vi "Axis Page.vi"() -> ()   [LabVIEW 2017, in "3D Plot.lvclass"]
uses:
  <vilib>/Math Plots/3D Math Plots/3D Plot/3D Plot/3D Plot.lvclass
  <vilib>/Math Plots/3D Math Plots/3D Plot/3D Plot/Typedef/Axis Property.ctl
  <vilib>/Math Plots/3D Math Plots/3D Plot/3D Plot/Typedef/Caption Property.ctl
  <vilib>/Math Plots/3D Math Plots/3D Plot/3D Plot/Typedef/Label Property.ctl
  <vilib>/Math Plots/3D Math Plots/3D Plot/3D Plot/Typedef/Range Property.ctl
  <vilib>/Math Plots/3D Math Plots/3D Plot/3D Plot/Typedef/Range Clusters.ctl
  <vilib>/Math Plots/3D Math Plots/3D Plot/3D Plot/Typedef/Grid Property.ctl
  <vilib>/Math Plots/3D Math Plots/3D Plot/3D Plot/Typedef/Tick Property.ctl
  <vilib>/Math Plots/3D Math Plots/3D Plot/3D Plot/Typedef/Dialog State.ctl
  <vilib>/Math Plots/3D Math Plots/3D Plot/3D Plot/Typedef/Temp Scene State.ctl
  <vilib>/Math Plots/3D Math Plots/3D Plot/3D Plot/Typedef/Temp Scene Property Action.ctl
panel:
  in  "Active Axis":u16(ring) caption="Active axis" items=["X Axis", "Y Axis", "Z Axis"]
  in  "Range Logarithm":bool caption="Range logarithm"
  in  "Marker Size":u16=1 caption="Size" min=1 step=1
  in  "Name Label Size":u16=1 caption="Size" min=1 step=1
  in  "Name Label Text":string caption="Text"
  in  "Marker Color":u32(colorbox) caption="Color"
  in  "Name Label Color":u32(colorbox) caption="Color"
  in  "Major Grid Color":u32(colorbox) caption="Major grid color"
  in  "Minor Grid Color":u32(colorbox) caption="Minor grid color"
  in  "Major Tick Color":u32(colorbox) caption="Major tick color"
  in  "Minor Tick Color":u32(colorbox) caption="Minor tick color"
  in  "Name Label Normal Visible":bool caption="Name label normal visible"
  in  "Name Label Opposite Visible":bool caption="Name label opposite visible"
  in  "Marker Normal Visible":bool caption="Marker normal visible"
  in  "Marker Opposite Visible":bool caption="Marker opposite visible"
  in  "Major Grid Visible":bool caption="Major grid visible"
  in  "Minor Grid Visible":bool caption="Minor grid visible"
  in  "Major Tick Visible":bool caption="Major tick visible"
  in  "Minor Tick Visible":bool caption="Major tick visible"
  in  "Major Tick Count":u16=1 caption="Major tick count" min=1 step=1
  in  "Minor Tick Count":u16=1 caption="Minor tick count" min=1 step=1
  in  "Range Auto Scale":bool caption="Range auto scale"
  in  "Range Inverted":bool caption="Range inverted"
  in  "Range Minimum":sgl caption="Minimum"
  in  "Range Maximum":sgl caption="Maximum"
  in  "Event Registration":refnum<event-registration>
  out "Axis Property Out":T1
  in  "Axis Property In":T1
  # "Axis"
  # "Name Label"
  # "Marker"
  # "Range"
  # "Grid"
  # "Tick"
  # "Tick Spacing"
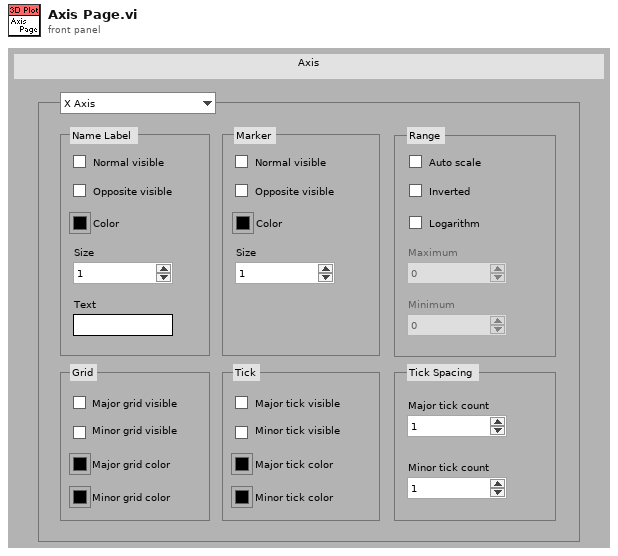
[diagram p1: front panel]
types:
  T1 = typedef "3D Plot.lvclass/Axis Property.ctl" = cluster{"Caption Property":T2, "Label Property":T3, "Range Property":T4, "Grid Property":T6, "Ticks Property":T7}
  T2 = typedef "3D Plot.lvclass/Caption Property.ctl" = cluster{"Show Caption":cluster{"Show Normal X Caption":bool, "Show Normal Y Caption":bool, "Show Normal Z Caption":bool, "Show Opposite X Caption":bool, "Show Opposite Y Caption":bool, "Show Opposite Z Caption":bool}, "Caption Color":cluster{"Caption Color X":u32, "Caption Color Y":u32, "Caption Color Z":u32}, "Caption Size":cluster{"Caption Size X":u16, "Caption Size Y":u16, "Caption Size Z":u16}, "Caption String":cluster{"Caption X":string, "Caption Y":string, "Caption Z ":string}}
  T3 = typedef "3D Plot.lvclass/Label Property.ctl" = cluster{"Show Label":cluster{"Show Normal X Label":bool, "Show Normal Y Label":bool, "Show Normal Z Label":bool, "Show Opposite X Label":bool, "Show Opposite Y Label":bool, "Show Opposite Z Label":bool}, "Label Color":cluster{"Label Color X":u32, "Label Color Y":u32, "Label Color Z":u32}, "Label Size":cluster{"Label Size X":u16, "Label Size Y":u16, "Labe Size Z":u16}}
  T4 = typedef "3D Plot.lvclass/Range Property.ctl" = cluster{"Range Cluster":T5, "Auto Range":cluster{"Auto Range X":bool, "Auto Range Y":bool, "Auto Range Z":bool}, "Inverted":cluster{"Inverted X":bool, "Inverted Y":bool, "Inverted Z":bool}, "Logarithm":cluster{"Logarithm X":bool, "Logarithm Y":bool, "Logarithm Z":bool}}
  T5 = typedef "3D Plot.lvclass/Range Clusters.ctl" = cluster{"X Range":cluster{"Max X":sgl, "Min X":sgl}, "Y Range":cluster{"Max Y":sgl, "Min Y":sgl}, "Z Range":cluster{"Max Z":sgl, "Min Z":sgl}}
  T6 = typedef "3D Plot.lvclass/Grid Property.ctl" = cluster{"Major Grid Visible":cluster{"Draw Major Grid X":bool, "Draw Major Grid Y":bool, "Draw Major Grid Z":bool}, "Major Grid Color":cluster{"Major Grid Color X":u32, "Major Grid Color Y":u32, "Major Grid Color Z":u32}, "Minor Grid Visible":cluster{"Draw Minor Grid X":bool, "Draw Minor Grid Y":bool, "Draw Minor Grid Z":bool}, "Minor Grid Color":cluster{"Minor Grid Color X":u32, "Minor Grid Color Y":u32, "Minor Grid Color Z":u32}}
  T7 = typedef "3D Plot.lvclass/Tick Property.ctl" = cluster{"Major Tick Visible":cluster{"Draw Major Tick X":bool, "Draw Major Tick Y":bool, "Draw Major Tick Z":bool}, "Major Tick Color":cluster{"Major Tick Color X":u32, "Major Tick Color Y":u32, "Major Tick Color Z":u32}, "Major Count":cluster{"Major Count X":u16, "Major Count Y":u16, "Major Count Z":u16}, "Minor Tick Visible":cluster{"Draw Minor Tick X":bool, "Draw Minor Tick Y":bool, "Draw Minor Tick Z":bool}, "Minor Tick Color":cluster{"Minor Tick Color X":u32, "Minor Tick Color Y":u32, "Minor Tick Color Z":u32}, "Minor Count":cluster{"Minor Count X":u16, "Minor Count Y":u16, "Minor Count Z":u16}}
  T8 = typedef "3D Plot.lvclass/Dialog State.ctl" = enum16{"Initialize", "Read Porperty", "Write Property", "Idle", "Exit"}
  T9 = typedef "3D Plot.lvclass/Axis Property Array Element.ctl" = cluster{"Caption":string, "Caption Size":u16, "Caption Color":u32, "Show Normal Caption":bool, "Show Opposite Caption":bool, "Label Size":u16, "Label Color":u32, "Show Normal Label":bool, "Show Opposite Label":bool, "Auto Range":bool, "Inverted":bool, "Logarithm":bool, "Max":sgl, "Min":sgl, "Draw Major Grid":bool, "Major Grid Color":u32, "Draw Minor Grid":bool, "Minor Grid Color":u32, "Major Count":u16, "Draw Major Tick":bool, "Major Tick Color":u32, "Minor Count":u16, "Draw Minor Tick":bool, "Minor Tick Color":u32}
  T10 = typedef "3D Plot.lvclass/Temp Scene State.ctl" = enum16{"Create", "Update Scene", "Get Plot Representation", "Destory"}
  T11 = typedef "3D Plot.lvclass/Temp Scene Property Action.ctl" = enum16{"Graph Property", "Light Property", "Axis Property", "Value Pair Property", "Format Property", "Cursor Property", "Plot Specific Property"}
  T12 = typedef "3D Plot.lvclass/Multiplot Representation.ctl" = cluster{"Plot Represention Array":T13[], "Max Range":T5}
  T13 = typedef "3D Plot.lvclass/Plot Representation.ctl" = cluster{"Plot ID":i32, "Plot Range":T5, "Mesh Data":T14, "Dimension":cluster{"X Dimension":i32, "Y Dimension":i32}, "Ramp Range":T5}
  T14 = typedef "3D Plot.lvclass/Mesh Data.ctl" = cluster{"Index Array":u32[], "Vertex Array":cluster{"X":sgl, "Y":sgl, "Z":sgl}[], "Normal Array":cluster{"X":sgl, "Y":sgl, "Z":sgl}[], "Color Index Array":i32[]}
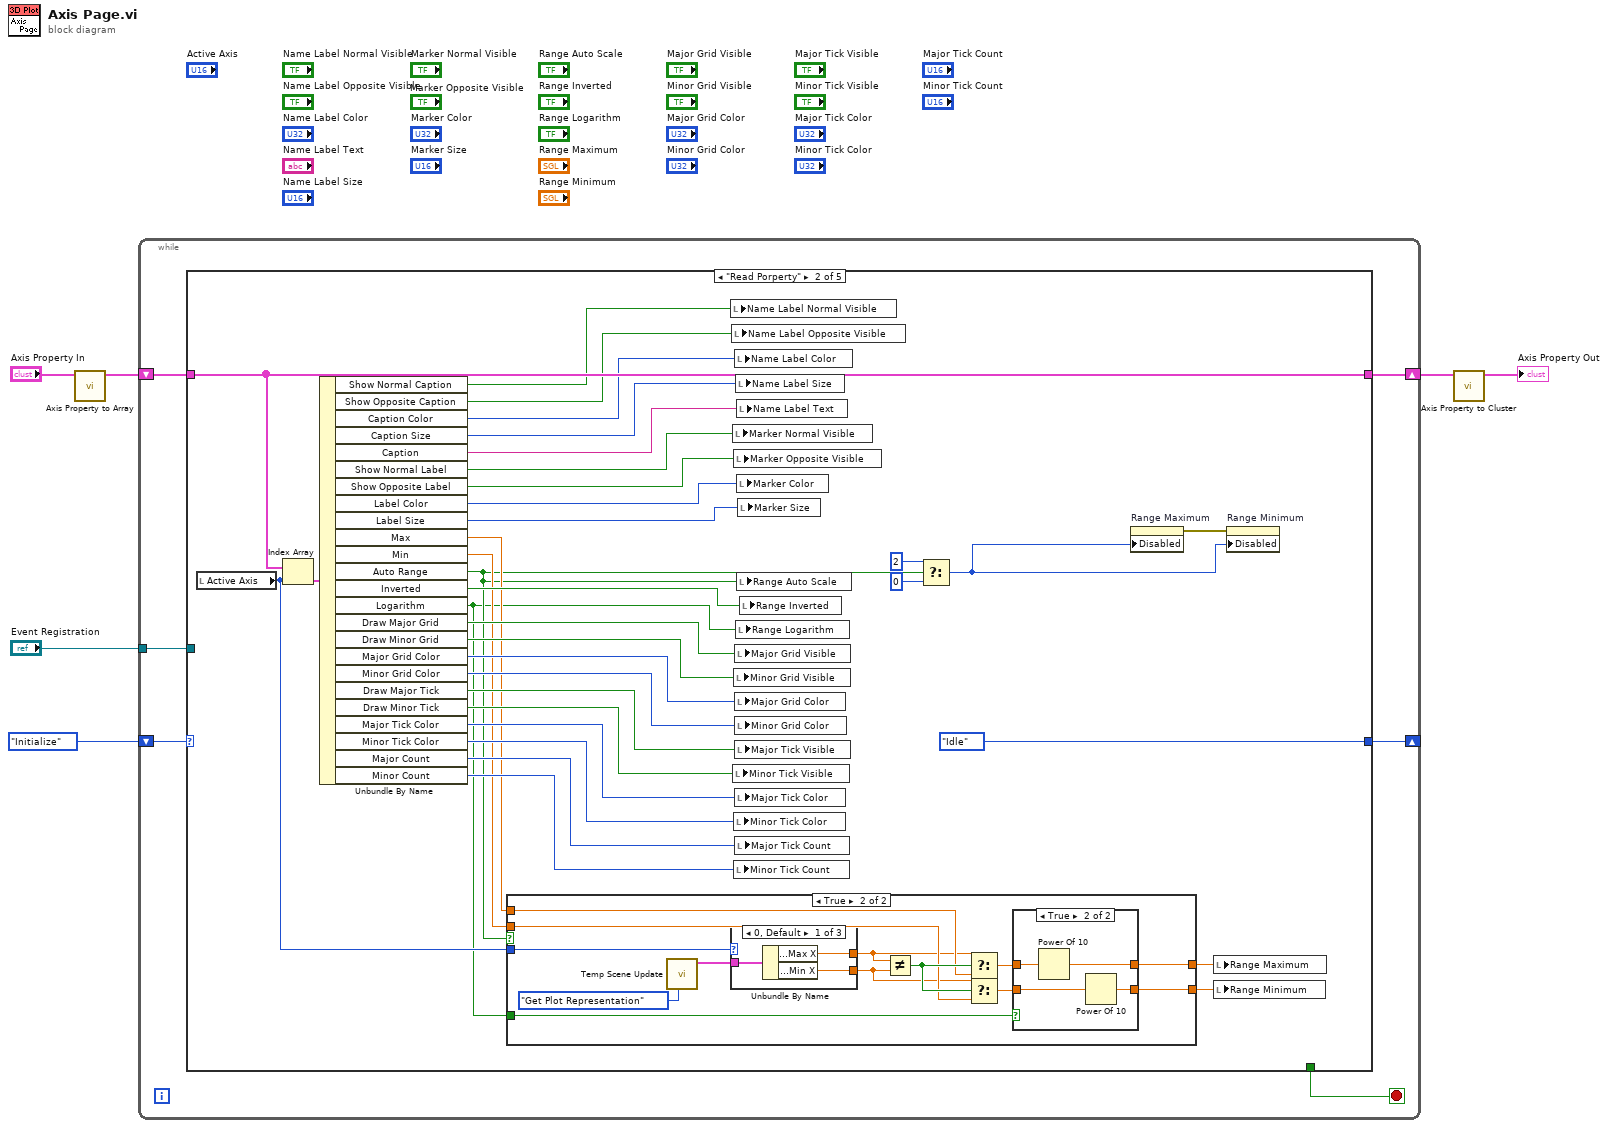
[diagram p0: block diagram]
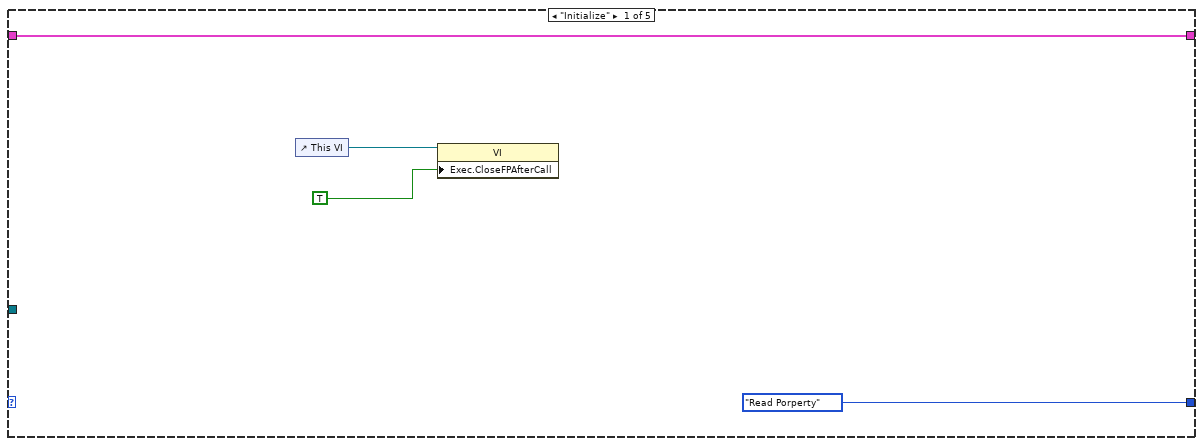
[diagram p2: hidden frame]
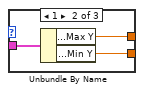
[diagram p5: hidden frame]
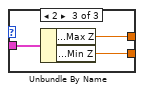
[diagram p6: hidden frame]
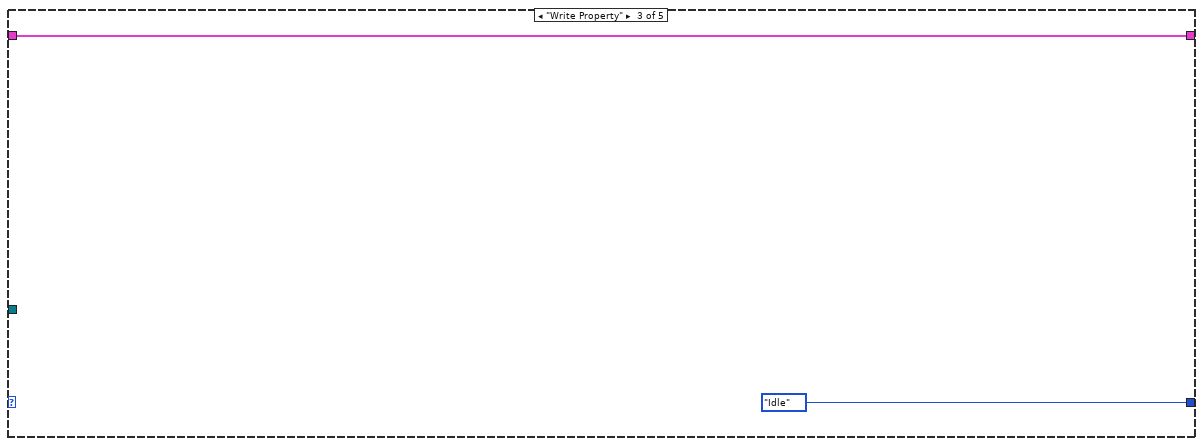
[diagram p7: hidden frame]
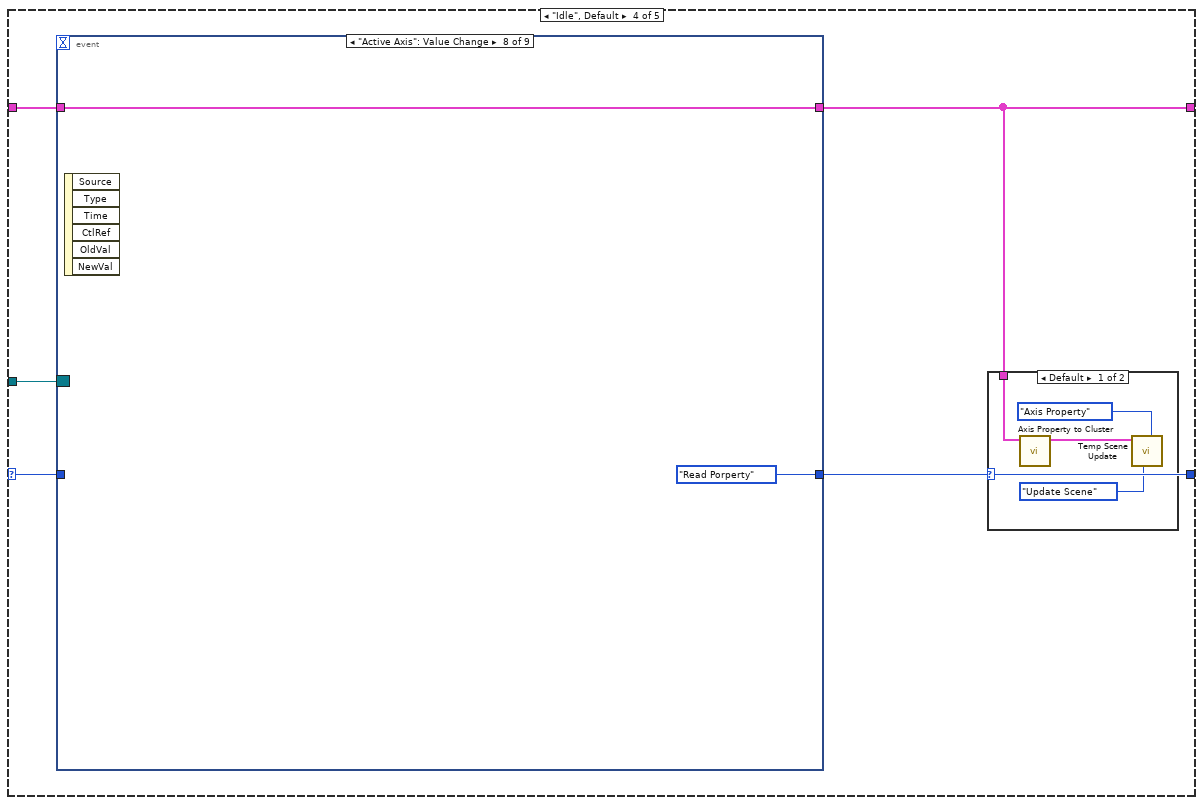
[diagram p8: hidden frame]
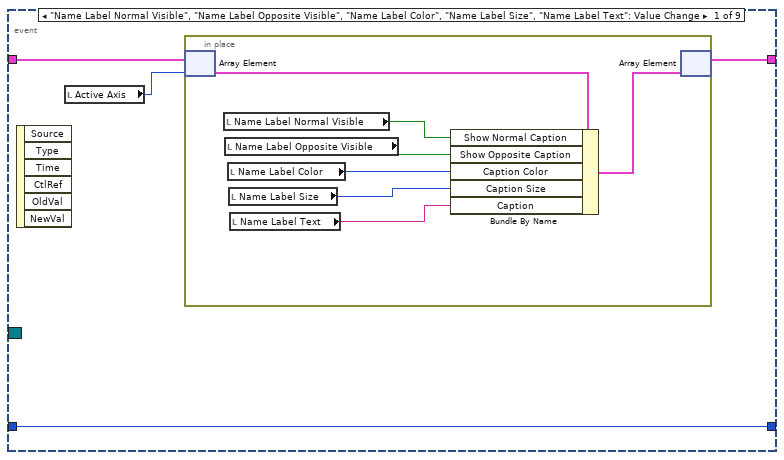
[diagram p10: hidden frame]
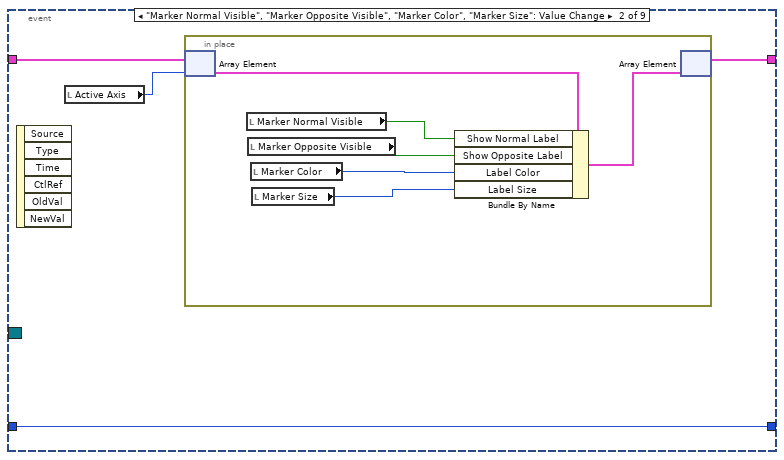
[diagram p11: hidden frame]
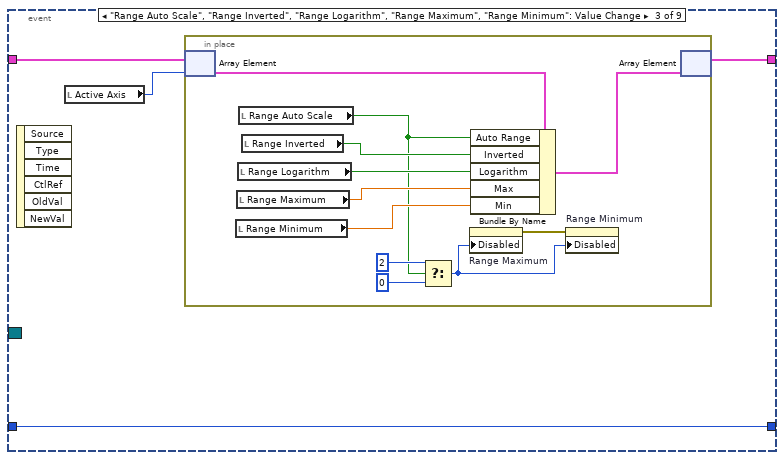
[diagram p12: hidden frame]
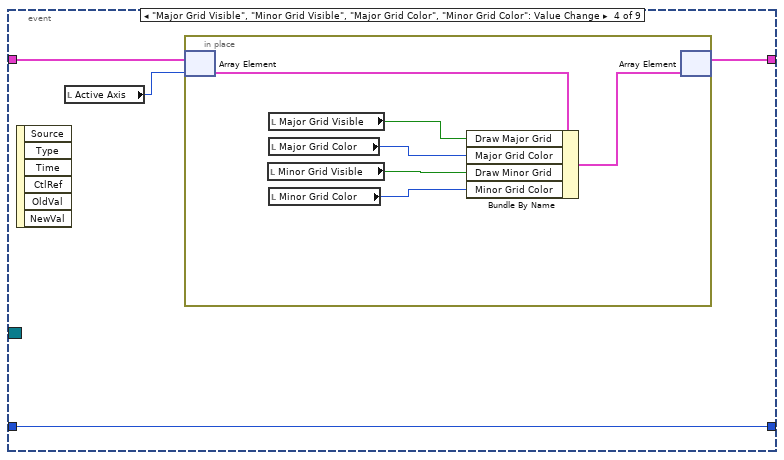
[diagram p13: hidden frame]
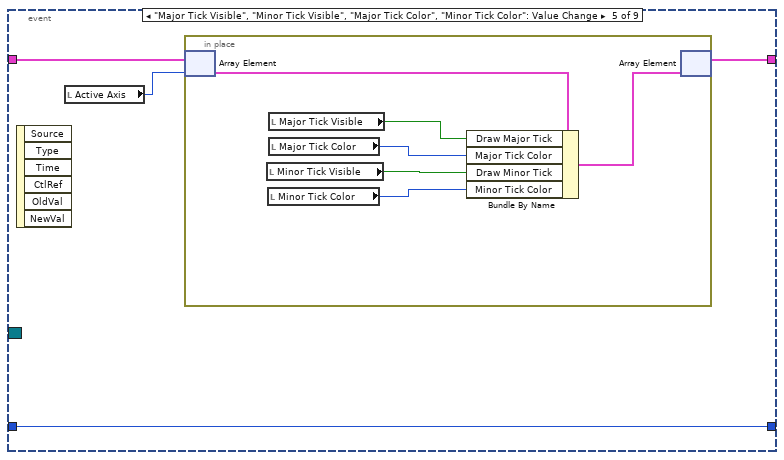
[diagram p14: hidden frame]
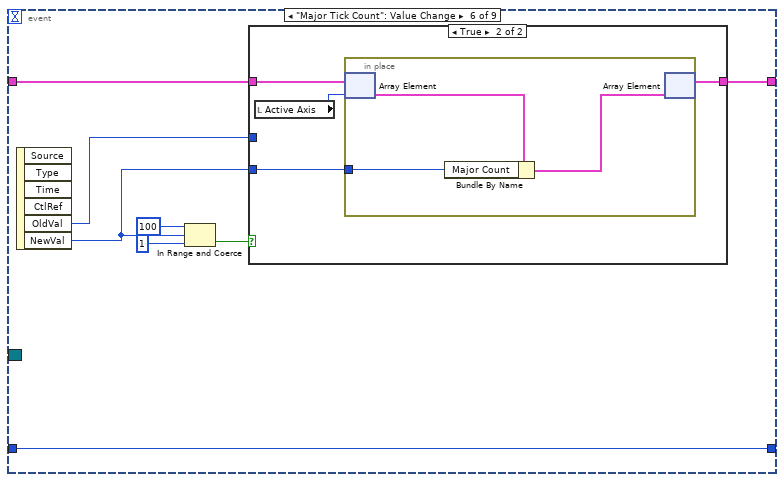
[diagram p15: hidden frame]
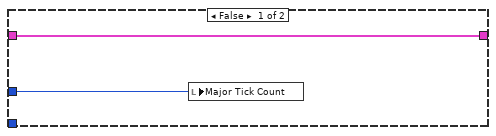
[diagram p16: hidden frame]
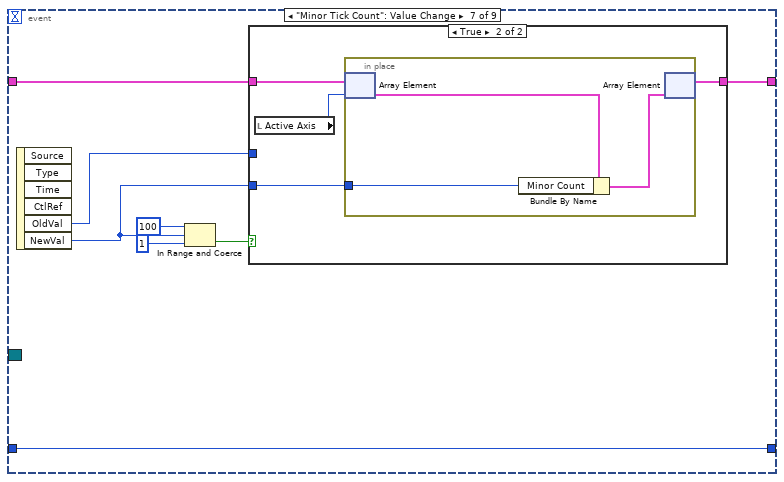
[diagram p17: hidden frame]
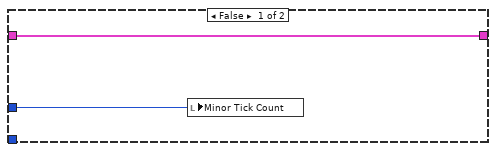
[diagram p18: hidden frame]
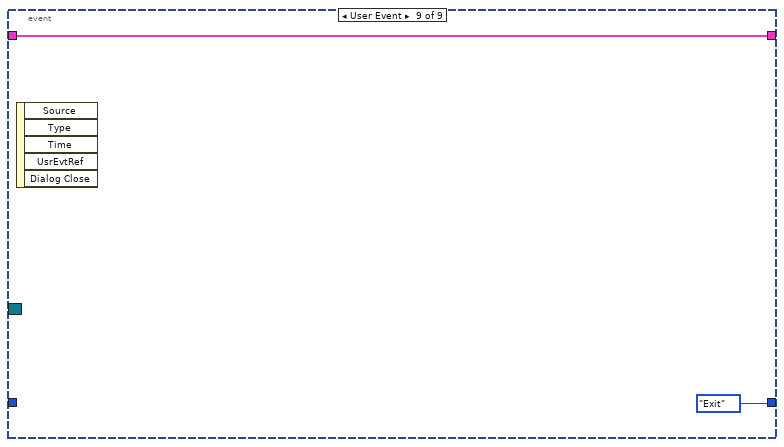
[diagram p19: hidden frame]
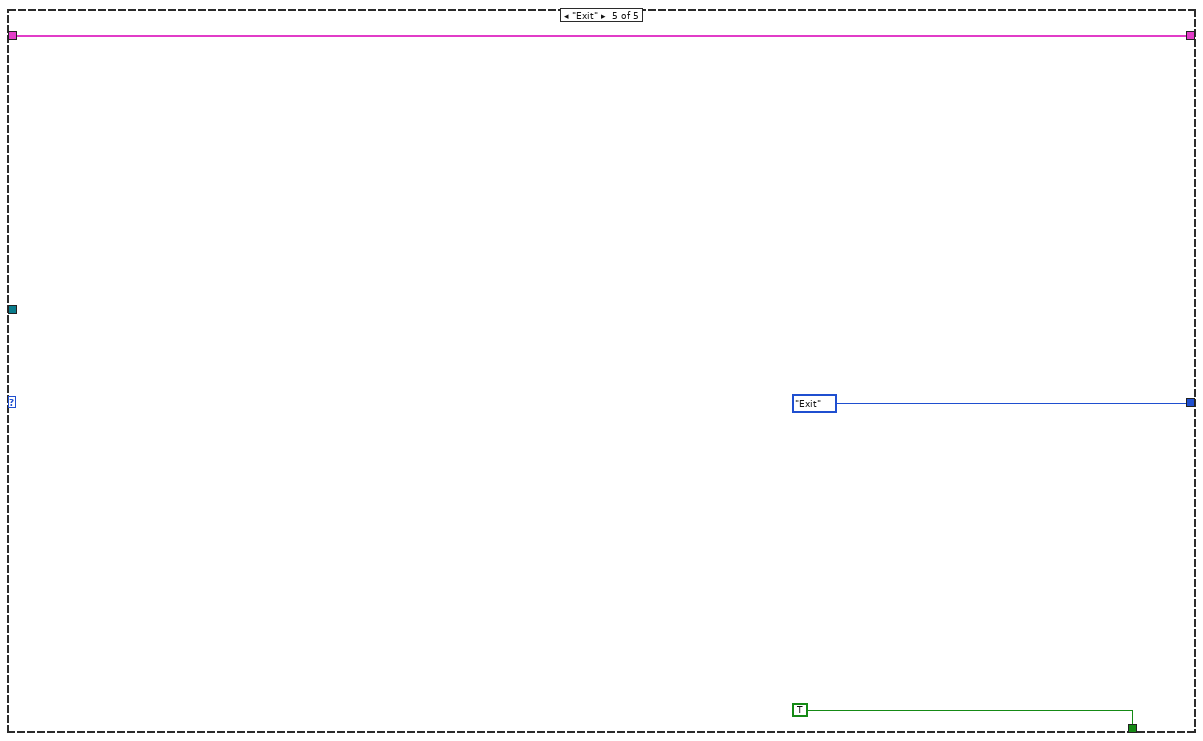
[diagram p20: hidden frame]
diagram:
  n1 = call <vilib>:"Axis Property to Array.vi"("Axis Property In"="Axis Property In") -> ("Axis Property Array Out"=w4:T9[])  [unwired: 10 out]
  n2 = while {
    shift-right: [w11] -> w3
    shift-left: w4 -> [w12]
    shift-right: [w7] -> _
    shift-left: Dialog_State."Initialize" -> [w10]
    tunnel: "Event Registration" -> [w8]
    stop <- w9 stop-if-true
    n3 = case shown="\"Read Porperty\"" w10 {
      selector: w10 -> [_ _ _ w85 _]
      tunnel: w12 -> [w15 w49 w81 w87 w186]
      tunnel: [w15 w49 w81 w84 w186] -> w11
      tunnel: [Dialog_State."Read Porperty" Dialog_State."Idle" Dialog_State."Idle" w83 Dialog_State."Exit"] -> w7
      tunnel: [_ _ _ _ TRUE] -> w9
      tunnel: w8 -> [_ _ _ w86 _]
      frame "Initialize" {
        n4 = control-ref of="This VI"() -> (w14:refnum<vi>)
        n5 = property class="VI"(reference=w14, "Exec.CloseFPAfterCall"=TRUE ("Execution:Close After Call")) -> ()  [unwired: 1 in, 2 out]
      }
      frame "Read Porperty" {
        n6 = local read "Active Axis"() -> (w23:u16)
        n7 = Index Array(array=w49, index=w23) -> (element=w48:T9)
        n8 = Unbundle By Name(w48) -> ("Show Normal Caption"=w47:bool, "Show Opposite Caption"=w46:bool, "Caption Color"=w45:u32, "Caption Size"=w44:u16, "Caption"=w43:string, "Show Normal Label"=w42:bool, "Show Opposite Label"=w41:bool, "Label Color"=w40:u32, "Label Size"=w39:u16, "Max"=w22:sgl, "Min"=w19:sgl, "Auto Range"=w18:bool, "Inverted"=w30:bool, "Logarithm"=w17:bool, "Draw Major Grid"=w36:bool, "Draw Minor Grid"=w38:bool, "Major Grid Color"=w37:u32, "Minor Grid Color"=w35:u32, "Draw Major Tick"=w31:bool, "Draw Minor Tick"=w32:bool, "Major Tick Color"=w33:u32, "Minor Tick Color"=w34:u32, "Major Count"=w29:u16, "Minor Count"=w28:u16)
        n9 = case shown="True" w18 {
          tunnel: w23 -> [_ w63]
          tunnel: w22 -> [w52 w60]
          tunnel: [w52 w54] -> w21
          tunnel: [w51 w56] -> w20
          tunnel: w19 -> [w51 w61]
          tunnel: w17 -> [_ w57]
          frame False {
          }
          frame True {
            n10 = call <vilib>:"Temp Scene Update.vi"("State"=Temp_Scene_State."Get Plot Representation") -> ("Multiplot Representation"=w64:T12)  [unwired: 5 in, 5 out]
            n11 = case shown="0, Default" w63 {
              tunnel: w64 -> [w74 w77 w80]
              tunnel: [w73 w76 w79] -> w59
              tunnel: [w72 w75 w78] -> w58
              frame 0, Default {
                n12 = Unbundle By Name(w74) -> ("Max Range.X Range.Max X"=w73:sgl, "Max Range.X Range.Min X"=w72:sgl)
              }
              frame 1 {
                n13 = Unbundle By Name(w77) -> ("Max Range.Y Range.Max Y"=w76:sgl, "Max Range.Y Range.Min Y"=w75:sgl)
              }
              frame 2 {
                n14 = Unbundle By Name(w80) -> ("Max Range.Z Range.Max Z"=w79:sgl, "Max Range.Z Range.Min Z"=w78:sgl)
              }
            }
            n15 = Not Equal?(x=w59, y=w58) -> (x != y?=w62:bool)
            n16 = Select(t=w59, s=w62, f=w60) -> (s? t:f=w53:sgl)
            n17 = Select(t=w58, s=w62, f=w61) -> (s? t:f=w55:sgl)
            n18 = case shown="True" w57 {
              tunnel: [w67 w69] -> w56
              tunnel: w55 -> [w67 w70]
              tunnel: [w66 w68] -> w54
              tunnel: w53 -> [w66 w71]
              frame False {
              }
              frame True {
                n19 = Power Of 10(x=w71) -> (10^x=w68:sgl)
                n20 = Power Of 10(x=w70) -> (10^x=w69:sgl)
              }
            }
          }
        }
        n21 = local write "Name Label Normal Visible"(w47) -> ()
        n22 = local write "Name Label Opposite Visible"(w46) -> ()
        n23 = local write "Marker Normal Visible"(w42) -> ()
        n24 = local write "Minor Tick Visible"(w32) -> ()
        n25 = local write "Marker Opposite Visible"(w41) -> ()
        n26 = local write "Minor Grid Visible"(w38) -> ()
        n27 = local write "Minor Tick Color"(w34) -> ()
        n28 = local write "Minor Tick Count"(w28) -> ()
        n29 = local write "Name Label Color"(w45) -> ()
        n30 = local write "Major Grid Visible"(w36) -> ()
        n31 = local write "Major Grid Color"(w37) -> ()
        n32 = local write "Minor Grid Color"(w35) -> ()
        n33 = local write "Major Tick Visible"(w31) -> ()
        n34 = local write "Major Tick Color"(w33) -> ()
        n35 = local write "Major Tick Count"(w29) -> ()
        n36 = local write "Name Label Size"(w44) -> ()
        n37 = local write "Range Logarithm"(w17) -> ()
        n38 = local write "Name Label Text"(w43) -> ()
        n39 = local write "Marker Color"(w40) -> ()
        n40 = local write "Range Auto Scale"(w18) -> ()
        n41 = local write "Marker Size"(w39) -> ()
        n42 = local write "Range Inverted"(w30) -> ()
        n43 = Select(t=u8 2 ("Disabled"), s=w18, f=u8 0 ("Disabled")) -> (s? t:f=w25:u8)
        n44 = property on="Range Maximum" class="DigNum (strict)"("Disabled"=w25) -> (error out=w24:errorcluster)  [unwired: 2 in, 1 out]
        n45 = local write "Range Maximum"(w21) -> ()
        n46 = local write "Range Minimum"(w20) -> ()
        n47 = property on="Range Minimum" class="DigNum (strict)"(error in=w24, "Disabled"=w25) -> ()  [unwired: 1 in, 2 out]
      }
      frame "Write Property" {
      }
      frame "Idle", Default {
        n48 = event shown="[7] \"Active Axis\": Value Change" {
          selector: w86 -> [_ _ _ _ _ _ _ _ _]
          dyn-events: _ -> [_ _ _ _ _ _ _ _ _]
          timeout: _ -> [_ _ _ _ _ _ _ _ _]
          tunnel: w87 -> [w95 w106 w116 w131 w141 w153 w169 w183 w185]
          tunnel: [w94 w105 w115 w130 w140 w154 w168 w183 w185] -> w84
          tunnel: [w92 w103 w113 w128 w138 w155 w165 Dialog_State."Read Porperty" Dialog_State."Exit"] -> w83
          tunnel: w85 -> [w92 w103 w113 w128 w138 w155 w165 _ _]
          event "Name Label Normal Visible", "Name Label Opposite Visible", "Name Label Color", "Name Label Size", "Name Label Text": Value Change {
            n49 = event-data() -> ()  [unwired: 7 out]
            n50 = local read "Active Axis"() -> (w93:u16)
            n51 = in-place {
              n52 = in-place-array #1(w95, w93) -> (w102:T9)
              n53 = local read "Name Label Normal Visible"() -> (w96:bool)
              n54 = local read "Name Label Opposite Visible"() -> (w97:bool)
              n55 = local read "Name Label Color"() -> (w98:u32)
              n56 = local read "Name Label Size"() -> (w99:u16)
              n57 = local read "Name Label Text"() -> (w100:string)
              n58 = Bundle By Name(cluster=w102, "Show Normal Caption"=w96, "Show Opposite Caption"=w97, "Caption Color"=w98, "Caption Size"=w99, "Caption"=w100) -> (w101:T9)
              n59 = in-place-array #1(w101) -> (w94:T9[])  [unwired: 1 out]
            }
          }
          event "Marker Normal Visible", "Marker Opposite Visible", "Marker Color", "Marker Size": Value Change {
            n60 = event-data() -> ()  [unwired: 7 out]
            n61 = local read "Active Axis"() -> (w104:u16)
            n62 = in-place {
              n63 = in-place-array #2(w106, w104) -> (w112:T9)
              n64 = local read "Marker Normal Visible"() -> (w107:bool)
              n65 = local read "Marker Opposite Visible"() -> (w108:bool)
              n66 = local read "Marker Color"() -> (w109:u32)
              n67 = local read "Marker Size"() -> (w110:u16)
              n68 = Bundle By Name(cluster=w112, "Show Normal Label"=w107, "Show Opposite Label"=w108, "Label Color"=w109, "Label Size"=w110) -> (w111:T9)
              n69 = in-place-array #2(w111) -> (w105:T9[])  [unwired: 1 out]
            }
          }
          event "Range Auto Scale", "Range Inverted", "Range Logarithm", "Range Maximum", "Range Minimum": Value Change {
            n70 = event-data() -> ()  [unwired: 7 out]
            n71 = local read "Active Axis"() -> (w114:u16)
            n72 = in-place {
              n73 = in-place-array #3(w116, w114) -> (w127:T9)
              n74 = local read "Range Minimum"() -> (w125:sgl)
              n75 = local read "Range Maximum"() -> (w124:sgl)
              n76 = local read "Range Logarithm"() -> (w122:bool)
              n77 = local read "Range Auto Scale"() -> (w117:bool)
              n78 = local read "Range Inverted"() -> (w123:bool)
              n79 = Select(t=u8 2 ("Disabled"), s=w117, f=u8 0 ("Disabled")) -> (s? t:f=w119:u8)
              n80 = property on="Range Maximum" class="DigNum (strict)"("Disabled"=w119) -> (error out=w118:errorcluster)  [unwired: 2 in, 1 out]
              n81 = Bundle By Name(cluster=w127, "Auto Range"=w117, "Inverted"=w123, "Logarithm"=w122, "Max"=w124, "Min"=w125) -> (w126:T9)
              n82 = property on="Range Minimum" class="DigNum (strict)"(error in=w118, "Disabled"=w119) -> ()  [unwired: 1 in, 2 out]
              n83 = in-place-array #3(w126) -> (w115:T9[])  [unwired: 1 out]
            }
          }
          event "Major Grid Visible", "Minor Grid Visible", "Major Grid Color", "Minor Grid Color": Value Change {
            n84 = event-data() -> ()  [unwired: 7 out]
            n85 = local read "Active Axis"() -> (w129:u16)
            n86 = in-place {
              n87 = in-place-array #4(w131, w129) -> (w137:T9)
              n88 = local read "Minor Grid Visible"() -> (w134:bool)
              n89 = local read "Major Grid Visible"() -> (w132:bool)
              n90 = local read "Major Grid Color"() -> (w133:u32)
              n91 = local read "Minor Grid Color"() -> (w135:u32)
              n92 = Bundle By Name(cluster=w137, "Draw Major Grid"=w132, "Major Grid Color"=w133, "Draw Minor Grid"=w134, "Minor Grid Color"=w135) -> (w136:T9)
              n93 = in-place-array #4(w136) -> (w130:T9[])  [unwired: 1 out]
            }
          }
          event "Major Tick Visible", "Minor Tick Visible", "Major Tick Color", "Minor Tick Color": Value Change {
            n94 = event-data() -> ()  [unwired: 7 out]
            n95 = local read "Active Axis"() -> (w139:u16)
            n96 = in-place {
              n97 = in-place-array #5(w141, w139) -> (w147:T9)
              n98 = local read "Minor Tick Visible"() -> (w144:bool)
              n99 = local read "Minor Tick Color"() -> (w145:u32)
              n100 = local read "Major Tick Visible"() -> (w142:bool)
              n101 = local read "Major Tick Color"() -> (w143:u32)
              n102 = Bundle By Name(cluster=w147, "Draw Major Tick"=w142, "Major Tick Color"=w143, "Draw Minor Tick"=w144, "Minor Tick Color"=w145) -> (w146:T9)
              n103 = in-place-array #5(w146) -> (w140:T9[])  [unwired: 1 out]
            }
          }
          event "Major Tick Count": Value Change {
            n104 = event-data() -> ("OldVal"=w148:u16, "NewVal"=w149:u16)  [unwired: 5 out]
            n105 = In Range and Coerce(upper limit=u16 100, x=w149, lower limit=u16 1) -> (In Range?=w150:bool)  [unwired: 1 out]
            n106 = case shown="True" w150 {
              tunnel: [w157 w161] -> w154
              tunnel: w153 -> [w157 w160]
              tunnel: w149 -> [_ w158]
              tunnel: w148 -> [w156 _]
              frame False {
                n107 = local write "Major Tick Count"(w156) -> ()
              }
              frame True {
                n108 = local read "Active Axis"() -> (w159:u16)
                n109 = in-place {
                  in-place-border: w158 -> [w162]
                  n110 = in-place-array #6(w160, w159) -> (w164:T9)
                  n111 = Bundle By Name(cluster=w164, "Major Count"=w162) -> (w163:T9)
                  n112 = in-place-array #6(w163) -> (w161:T9[])  [unwired: 1 out]
                }
              }
            }
          }
          event "Minor Tick Count": Value Change {
            n113 = event-data() -> ("OldVal"=w166:u16, "NewVal"=w167:u16)  [unwired: 5 out]
            n114 = In Range and Coerce(upper limit=u16 100, x=w167, lower limit=u16 1) -> (In Range?=w170:bool)  [unwired: 1 out]
            n115 = case shown="True" w170 {
              tunnel: [w174 w178] -> w168
              tunnel: w169 -> [w174 w177]
              tunnel: w167 -> [_ w175]
              tunnel: w166 -> [w173 _]
              frame False {
                n116 = local write "Minor Tick Count"(w173) -> ()
              }
              frame True {
                n117 = local read "Active Axis"() -> (w176:u16)
                n118 = in-place {
                  in-place-border: w175 -> [w179]
                  n119 = in-place-array #7(w177, w176) -> (w181:T9)
                  n120 = Bundle By Name(cluster=w181, "Minor Count"=w179) -> (w180:T9)
                  n121 = in-place-array #7(w180) -> (w178:T9[])  [unwired: 1 out]
                }
              }
            }
          }
          event "Active Axis": Value Change {
            n122 = event-data() -> ()  [unwired: 7 out]
          }
          event User Event {
            n123 = event-data() -> ()  [unwired: 6 out]
          }
        }
        n124 = case shown="Default" w83 {
          tunnel: w84 -> [w90 _]
          frame Default {
            n125 = call <vilib>:"Axis Property to Cluster.vi"("Axis Property Array In"=w90) -> ("Axis Property Out"=w89:T1)  [unwired: 10 out]
            n126 = call <vilib>:"Temp Scene Update.vi"("Property Name"=Temp_Scene_Property_Action."Axis Property", "State"=Temp_Scene_State."Update Scene", "Property In"=w89) -> ()  [unwired: 3 in, 6 out]
          }
          frame "Exit" {
          }
        }
      }
      frame "Exit" {
      }
    }
  }
  n127 = call <vilib>:"Axis Property to Cluster.vi"("Axis Property Array In"=w3) -> ("Axis Property Out"=→"Axis Property Out":T1)  [unwired: 10 out]
